vi "focusmapping.vi"(4 "Current Y Position":dbl, 6 "Current X Position":dbl, 9 "Z Locations":dbl[](array[numeric]), 10 "Y Locations":dbl[](array[numeric]), 11 "X Locations":dbl[](array[numeric])) -> (3 "MoveTo Z":dbl)   [LabVIEW 2023]
uses:
  <vilib>/gmath/interp.llb/Interpolate 2D Scattered (1D).vi
  <vilib>/gmath/NI_AAL_Interpolation.lvlib
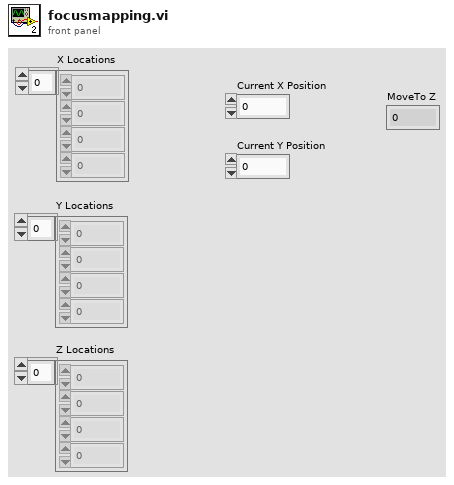
[diagram p1: front panel]
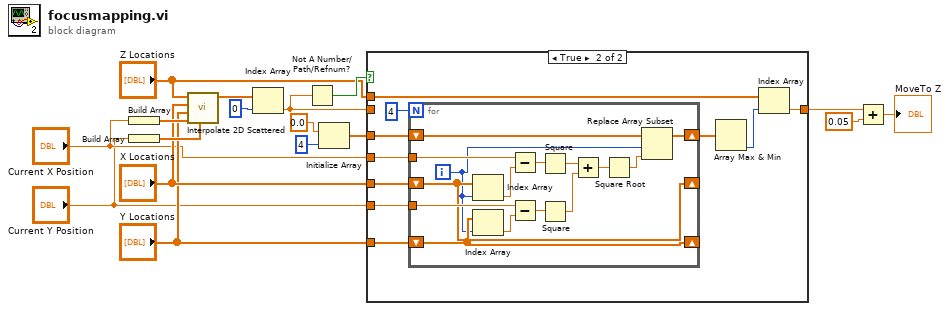
[diagram p0: block diagram]
diagram:
  n1 = Build Array("Current X Position") -> (w17:dbl[])
  n2 = Build Array("Current Y Position") -> (w16:dbl[])
  n3 = call-poly <vilib>:"Interpolate 2D Scattered.vi"("Yi"=w16, "Xi"=w17, "Y"="Y Locations", "X"="X Locations", "Z"="Z Locations") -> ("Zi"=w15:dbl[])  [unwired: 5 in, 1 out]
  n4 = Index Array(array=w15, index=0) -> (element=w12:dbl)
  n5 = Not A Number/Path/Refnum?(number/path/refnum=w12) -> (NaN/Path/Refnum?=w13:bool)
  n6 = Initialize Array(0.0 ("element"), 4 ("dimension size")) -> (w7:dbl[])
  n7 = case shown="True" w13 {
    tunnel: w12 -> [w18 _]
    tunnel: [w18 w20] -> w3
    tunnel: "X Locations" -> [_ w27]
    tunnel: "Y Locations" -> [_ w26]
    tunnel: w7 -> [_ w25]
    tunnel: "Current X Position" -> [_ w24]
    tunnel: "Current Y Position" -> [_ w23]
    tunnel: "Z Locations" -> [_ w21]
    frame False {
    }
    frame True {
      n8 = for {
        N: 4 -> [_]
        shift-right: [w32] -> _
        shift-left: w27 -> [w32]
        shift-right: [w31] -> _
        shift-left: w26 -> [w31]
        shift-right: [w30] -> w19
        shift-left: w25 -> [w34]
        tunnel: w24 -> [w43]
        tunnel: w23 -> [w41]
        i -> [w29]
        n9 = Index Array(array=w32, index=w29) -> (element=w42:dbl)
        n10 = Index Array(array=w31, index=w29) -> (element=w40:dbl)
        n11 = Subtract(x=w43, y=w42) -> (x-y=w39:dbl)
        n12 = Subtract(x=w41, y=w40) -> (x-y=w38:dbl)
        n13 = Square(x=w39) -> (x^2=w37:dbl)
        n14 = Square(x=w38) -> (x^2=w36:dbl)
        n15 = Add(x=w37, y=w36) -> (x+y=w35:dbl)
        n16 = Square Root(x=w35) -> (sqrt(x)=w33:dbl)
        n17 = Replace Array Subset(array=w34, new element=w33, index=w29) -> (w30:dbl[])
      }
      n18 = Array Max & Min(array=w19) -> (min index (indices)=w22:i32)  [unwired: 3 out]
      n19 = Index Array(array=w21, index=w22) -> (element=w20:dbl)
    }
  }
  n20 = Add(x=w3, y=0.05) -> (x+y=→"MoveTo Z":dbl)
